vi "Configure Math.vi"   [LabVIEW 2020, in "Counter.lvlib" / "PICOTEST U62XXA series.lvlib"]
doc: "Configures post acquisition math operations."
uses:
  PICOTEST U62XXA series.lvlib
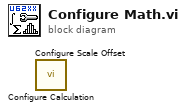
[diagram p0: block diagram]
diagram:
  n1 = call "Configure Calculation.vi"() -> ()  [unwired: 10 in, 2 out]
  n2 = call "Configure Scale Offset.vi"() -> ()  [unwired: 10 in, 2 out]
